vi "Send Command.vi"(8 "error in":errorcluster, 9 "Value":variant, 10 "Command":string, 11 "DIG_IO in":refnum<class "DIG_IO.lvclass">) -> (0 "error out":errorcluster, 3 "DIG_IO out":refnum<class "DIG_IO.lvclass">)   [LabVIEW 2019, in "DIG_IO.lvlib" / "DIG_IO.lvclass"]
uses:
  Library/DIG_IO.lvclass
  C:/Users/Public/Documents/Development/builds/Engine/Engine.lvlibp/Project/Engine.lvclass
  C:/Users/Public/Documents/Development/builds/Engine/Monitored Actor.lvlibp/Monitored Actor/Monitored Actor/Monitored Actor.lvclass
  DIG_IO Messages/Set by Name Msg/Set by Name Msg.lvclass/Set by Name Msg.ctl
  DIG_IO Messages/Toggle IO Enable Msg/Toggle IO Enable Msg.lvclass/Toggle IO Enable Msg.ctl
  DIG_IO Messages/Pulse Output Msg/Pulse Output Msg.lvclass/Pulse Output Msg.ctl
  DIG_IO Messages/Write Pulse Width Msg/Write Pulse Width Msg.lvclass/Write Pulse Width Msg.ctl
  builds/Engine/Engine.lvlibp/Accessors/Read Self Q.vi
  builds/Engine/Monitored Actor.lvlibp/Monitored Actor/Monitored Actor/Read Actor Label.vi
  <vilib>/Utility/error.llb/Error Cluster From Error Code.vi
  builds/Engine/Actor Framework.lvlibp/1abvi3w/vi.lib/ActorFramework/Message Enqueuer/Enqueue.vi
  builds/Engine/Actor Framework.lvlibp/1abvi3w/vi.lib/ActorFramework/Message Enqueuer/Message Enqueuer.lvclass
  <vilib>/ErrorRing/Error Ring.xnode
  DIG_IO Messages/Set by Name Msg/Set by Name Msg.lvclass
  DIG_IO Messages/Clear All Discretes Msg/Clear All Discretes Msg.lvclass
  DIG_IO Messages/Toggle IO Enable Msg/Toggle IO Enable Msg.lvclass
  DIG_IO Messages/Pulse Output Msg/Pulse Output Msg.lvclass
  DIG_IO Messages/Write Pulse Width Msg/Write Pulse Width Msg.lvclass
  builds/Engine/Engine.lvlibp/Project/Engine.lvclass
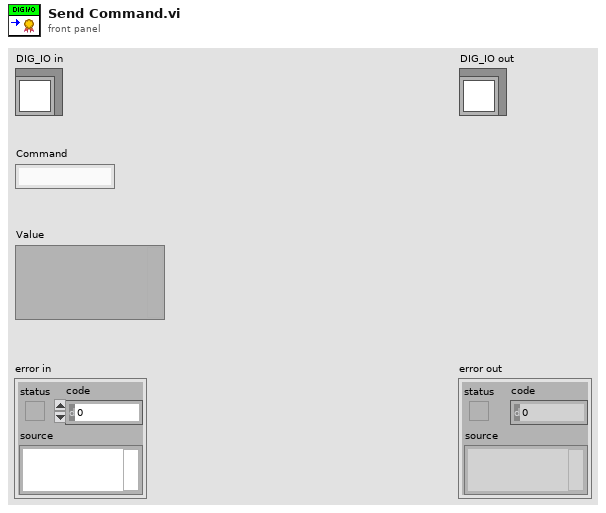
[diagram p1: front panel]
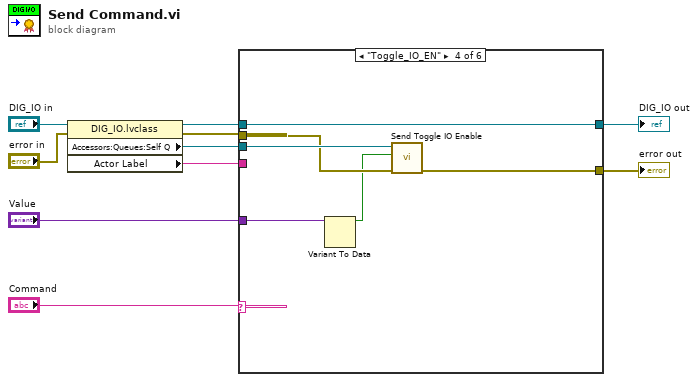
[diagram p0: block diagram]
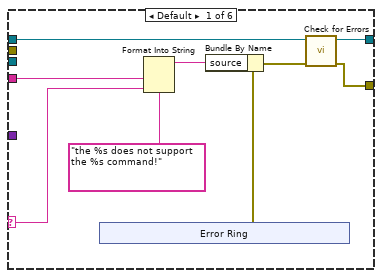
[diagram p2: hidden frame]
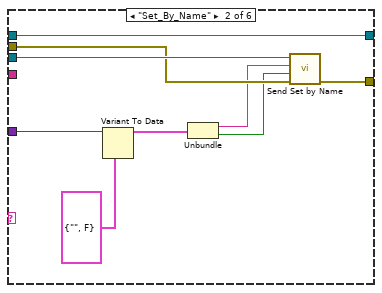
[diagram p3: hidden frame]
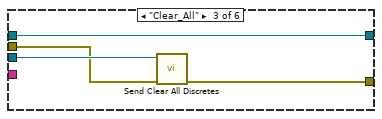
[diagram p4: hidden frame]
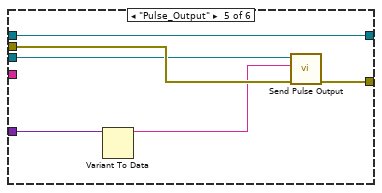
[diagram p5: hidden frame]
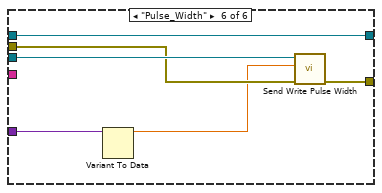
[diagram p6: hidden frame]
diagram:
  n1 = property class="DIG_IO.lvclass"(reference="DIG_IO in", error in="error in") -> (reference out=w7:refnum<class "DIG_IO.lvclass">, error out=w4:errorcluster, "Accessors:Queues:Self Q"=w5:refnum<class "Message Enqueuer.lvclass">, "Actor Label"=w1:string)
  n2 = case shown="\"Toggle_IO_EN\"" "Command" {
    selector: "Command" -> [w11 _ _ _ _ _]
    tunnel: "Value" -> [_ w30 _ w38 w47 w53]
    tunnel: w7 -> [w19 w32 w36 w42 w48 w54]
    tunnel: [w18 w32 w36 w42 w48 w54] -> w6
    tunnel: w5 -> [_ w31 w35 w41 w44 w52]
    tunnel: w4 -> [_ w29 w34 w40 w46 w51]
    tunnel: [w17 w26 w33 w39 w45 w50] -> w2
    tunnel: w1 -> [w12 _ _ _ _ _]
    frame Default {
      n3 = xnode "Error Ring"() -> ("error out"=w16:errorcluster)
      n4 = Format Into String(format string="the %s does not support the %s command!", w12, w11) -> (resulting string=w13:string)  [unwired: 2 in, 1 out]
      n5 = Bundle By Name(cluster=w16, "source"=w13) -> (w15:errorcluster)
      n6 = call "Check for Errors.vi"("error in"=w15, "Engine in"=w19) -> ("error out"=w17:errorcluster, "Engine out"=w18:refnum<class "DIG_IO.lvclass">)  [unwired: 8 in]
    }
    frame "Set_By_Name" {
      n7 = Variant To Data(type=cluster{"Name":string, "Value":bool} {"Name"="", "Value"=FALSE}, Variant=w30) -> (data=w28:cluster{"Name":string, "Value":bool})  [unwired: 1 in, 1 out]
      n8 = Unbundle(w28) -> ("Name"=w25:string, "Value"=w24:bool)
      n9 = call "Send Set by Name.vi"("error in (no error)"=w29, "Value"=w24, "Channel Name"=w25, "Message Enqueuer"=w31) -> ("error out"=w26:errorcluster)  [unwired: 6 in, 1 out]
    }
    frame "Clear_All" {
      n10 = call "Send Clear All Discretes.vi"("error in (no error)"=w34, "Message Enqueuer"=w35) -> ("error out"=w33:errorcluster)  [unwired: 8 in, 1 out]
    }
    frame "Toggle_IO_EN" {
      n11 = Variant To Data(Variant=w38) -> (data=w37:bool)  [unwired: 2 in, 1 out]
      n12 = call "Send Toggle IO Enable.vi"("error in (no error)"=w40, "IO_EN"=w37, "Message Enqueuer"=w41) -> ("error out"=w39:errorcluster)  [unwired: 7 in, 1 out]
    }
    frame "Pulse_Output" {
      n13 = Variant To Data(Variant=w47) -> (data=w43:string)  [unwired: 2 in, 1 out]
      n14 = call "Send Pulse Output.vi"("error in (no error)"=w46, "Target"=w43, "Message Enqueuer"=w44) -> ("error out"=w45:errorcluster)  [unwired: 7 in, 1 out]
    }
    frame "Pulse_Width" {
      n15 = Variant To Data(Variant=w53) -> (data=w49:dbl)  [unwired: 2 in, 1 out]
      n16 = call "Send Write Pulse Width.vi"("error in (no error)"=w51, "Period"=w49, "Message Enqueuer"=w52) -> ("error out"=w50:errorcluster)  [unwired: 7 in, 1 out]
    }
  }
  "error out" <- w2
  "DIG_IO out" <- w6
